vi "Write Transceiver Response.vi"(6 "overwrite on timeout (T)":bool, 8 "error in (no error)":errorcluster, 9 "timeout in ms (0)":i32, 10 "response":T1, 11 "Transceiver Interface in":refnum<class "Transceiver Interface.lvclass">) -> (0 "error out":errorcluster, 1 "timed out?":bool, 3 "Transceiver Interface out":refnum<class "Transceiver Interface.lvclass">)   [LabVIEW 2017, in "DSF Core.lvlib" / "Transceiver Interface.lvclass"]
uses:
  Transceiver Interface.lvclass
  C:/Git/DSF/Data Sharing Framework/Source/Core/Engine/Classes/Interfaces/Interface/Interface.lvclass
  Response Data.ctl
  Response.ctl
  Response Parameters.ctl
  Interface/RT FIFO Data 16B.ctl
  Interface/RT FIFO Payload 16B.ctl
  Interface/Interface.lvclass/Interface.ctl
  Debug/FIFO Flags/FIFO Flags.lvclass/FIFO Flags.ctl
  Interface/Write RT FIFO(16B).vi
  Interface/Get Debug Flags.vi
  Interface/Get Response FIFO.vi
  Debug/FIFO Flags/Get Infinite Timeouts.vi
  Interface/Errors.vi
  Interface/Response Timeout.vi
  Interface/Interface.lvclass
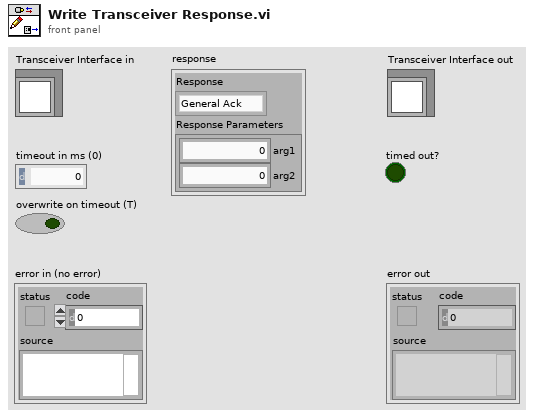
[diagram p1: front panel]
types:
  T1 = typedef "DSF Core.lvlib/Transceiver Interface.lvclass/Response Data.ctl" = cluster{"Response":T2, "Response Parameters":T3}
  T2 = typedef "DSF Core.lvlib/Transceiver Interface.lvclass/Response.ctl" = enum8{"General Ack", "Shutting Down"}
  T3 = typedef "DSF Core.lvlib/Transceiver Interface.lvclass/Response Parameters.ctl" = cluster{"arg1":u64, "arg2":u64}
  T4 = typedef "DSF Core.lvlib/Interface.lvclass/RT FIFO Data 16B.ctl" = cluster{"Command":u8, "Payload":T5}
  T5 = typedef "DSF Core.lvlib/Interface.lvclass/RT FIFO Payload 16B.ctl" = cluster{"arg1":u64, "arg2":u64}
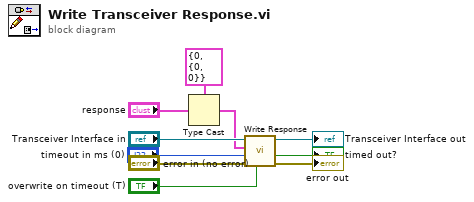
[diagram p0: block diagram]
diagram:
  n1 = Type Cast(type=T4 {"Command"=0, "Payload"={"arg1"=0, "arg2"=0}} ("element"), x="response") -> (*(type *) &x=w2:T4)
  n2 = call "Write Response.vi"("overwrite on timeout (T)"="overwrite on timeout (T)", "error in (no error)"="error in (no error)", "timeout in ms (0)"="timeout in ms (0)", "response"=w2, "Interface in"="Transceiver Interface in") -> ("error out"=→"error out":errorcluster, "timed out?"=→"timed out?":bool, "Interface out"=→"Transceiver Interface out":refnum<class "Transceiver Interface.lvclass">)  [unwired: 4 in]
